vi "BNO055 receive init.vi"(8 "error in (no error)":errorcluster) -> (0 "error out":errorcluster, 1 "element":dbl, 3 "rt fifo out":refnum<k33>)   [LabVIEW 2019]
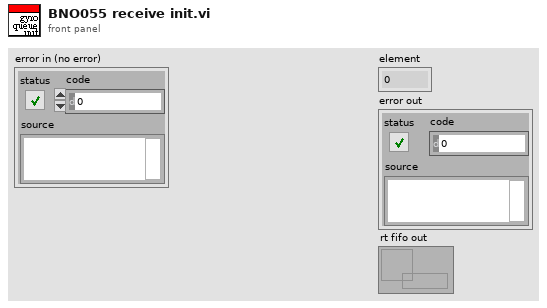
[diagram p1: front panel]
types:
  T1 = cluster{"read mode":enum16{"polling", "blocking"}, "write mode":enum16{"polling", "blocking"}}
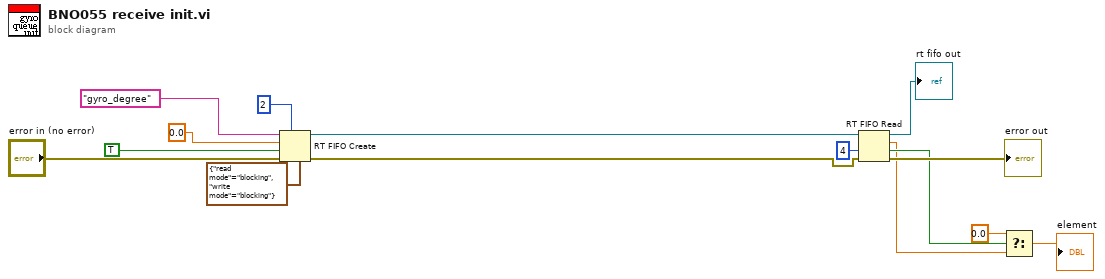
[diagram p0: block diagram]
diagram:
  n1 = RT FIFO Create(0:"gyro_degree" ("name (unnamed)"), 1:0.0, 2:TRUE ("create if not found? (T)"), 3:"error in (no error)", 4:u32 2 ("size (10)"), 7:T1 {"read mode"=enum."blocking", "write mode"=enum."blocking"} ("r/w modes (polling,polling)")) -> (8:w2:refnum<k33>, 11:w10:errorcluster)  [unwired: 2 in, 1 out]
  n2 = RT FIFO Read(0:w2, 2:4 ("timeout in ms (-1)"), 3:w10) -> (8:→"rt fifo out":refnum<k33>, 9:w3:dbl, 10:w7:bool, 11:→"error out":errorcluster)  [unwired: 1 in, 1 out]
  n3 = Select(t=0.0, s=w7, f=w3) -> (s? t:f=→"element":dbl)
